vi "Apply Theme To ActionButtons.vi"(7 "Override Root With (Empty)":string, 8 "Error In":errorcluster, 9 "Window Element":T1, 10 "ActionButtons Ref":refnum<vi>[](array[refnum]), 11 "Generic Theme in":refnum<class "Generic Theme.lvclass">) -> (0 "Error Out":errorcluster, 3 "Generic Theme out":refnum<class "Generic Theme.lvclass">)   [LabVIEW 2021, in "Appearance Actor.lvlib" / "Generic Theme.lvclass"]
doc: "Apply theme to <B>ActionButtons</B> (Bool Reference Array). <B>Window Element</B> enum tells where it is on the window. <B>Override Root With</B> allows to override styling used for main window components."
uses:
  Generic Theme.lvclass
  Typedefs/Window Element--enum.ctl
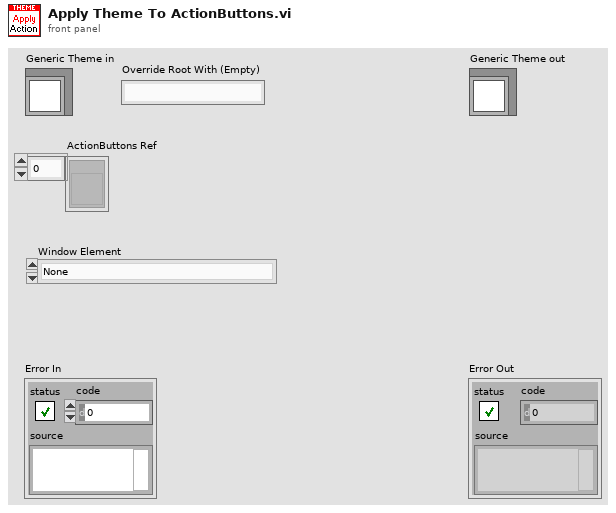
[diagram p1: front panel]
types:
  T1 = typedef "Appearance Actor.lvlib/Generic Theme.lvclass/Window Element--enum.ctl" = enum16{"None", "TitleBar", "SideMenu", "BodyPane"}
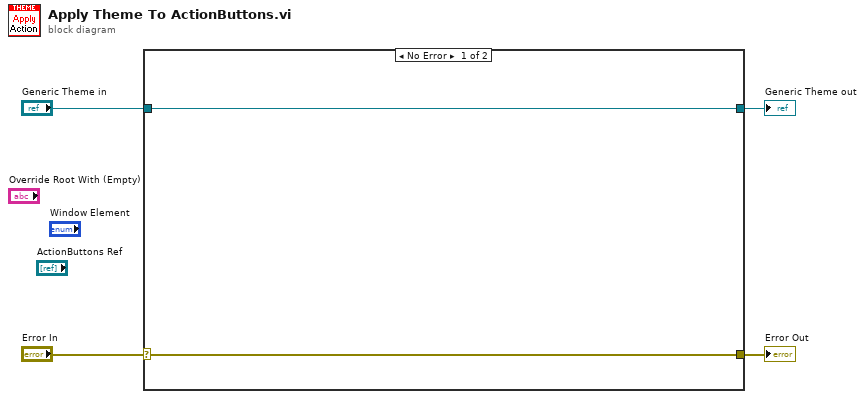
[diagram p0: block diagram]
diagram:
  n1 = case shown="No Error" "Error In" {
    selector: "Error In" -> [w5 w8]
    tunnel: [w5 w8] -> w3
    tunnel: [w6 w7] -> w1
    tunnel: "Generic Theme in" -> [w6 w7]
    frame No Error {
    }
    frame Error {
    }
  }
  "Error Out" <- w3
  "Generic Theme out" <- w1
